vi "Get Size with Offset.vi"(8 "error in (no error)":errorcluster, 11 "Channel Runtime in":refnum<class "Runtime.Channel.lvclass">) -> (0 "error out":errorcluster, 2 "size+offset in bytes":u64, 3 "Channel Runtime out":refnum<class "Runtime.Channel.lvclass">)   [LabVIEW 2016, in "Data Sharing Framework.Runtime.lvlib" / "Runtime.Channel.lvclass"]
uses:
  Runtime.Channel.lvclass
  Runtime.Channel.lvclass/Runtime.Channel.ctl
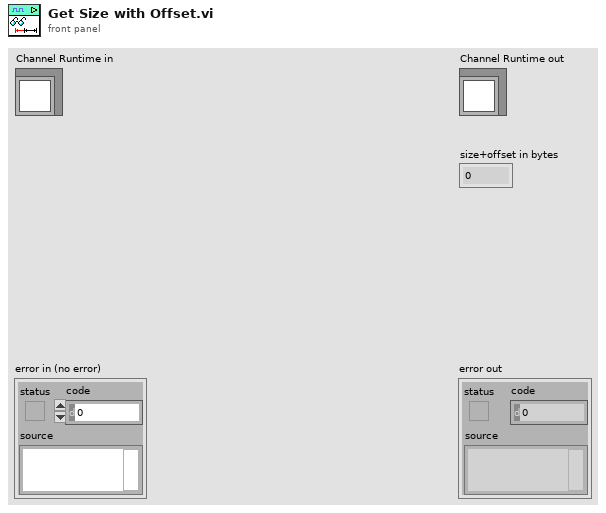
[diagram p1: front panel]
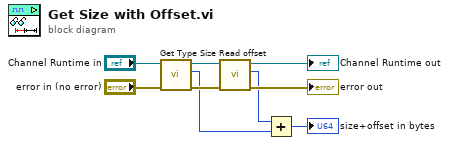
[diagram p0: block diagram]
diagram:
  n1 = call "Get Type Size.vi"("error in (no error)"="error in (no error)", "Channel Runtime in"="Channel Runtime in") -> ("error out"=w8:errorcluster, "size in bytes"=w6:u64, "Channel Runtime out"=w7:refnum<class "Runtime.Channel.lvclass">)  [unwired: 7 in]
  n2 = call "Read offset.vi"("error in (no error)"=w8, "Runtime.Channel in"=w7) -> ("error out"=→"error out":errorcluster, "offset"=w1:u64, "Runtime.Channel out"=→"Channel Runtime out":refnum<class "Runtime.Channel.lvclass">)  [unwired: 7 in]
  n3 = Add(x=w1, y=w6) -> (x+y=→"size+offset in bytes":u64)
